vi "Versioned UI Post-Build Action.vi"(5 "Files Generated by Build":path[](array[path]), 6 "Top Level/Always Included VIs":path[](array[path]), 7 "Destination Path":path, 8 "error in (no error)":errorcluster, 9 "Target Name":string, 10 "Build Specification Name":string, 11 "Project Path":path) -> (0 "error out":errorcluster)   [LabVIEW 2021, in "CIF Build Actions.lvlib"]
uses:
  CIF Build Actions.lvlib
  <vilib>/regexp/Match Regular Expression.xnode
  CIFConfigurationFile/CIF Configuration File.lvlib
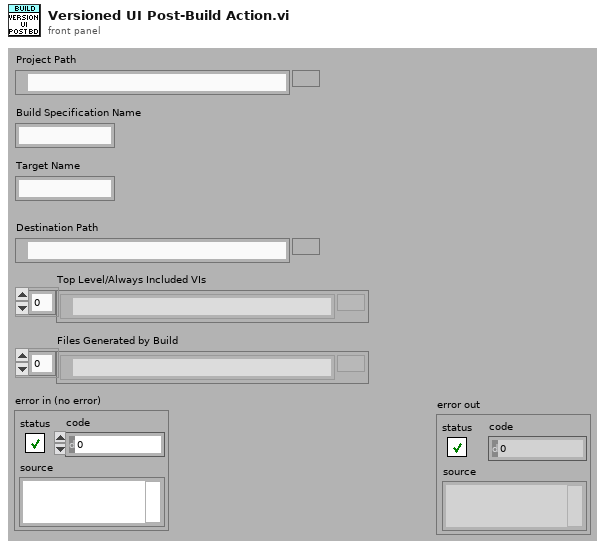
[diagram p1: front panel]
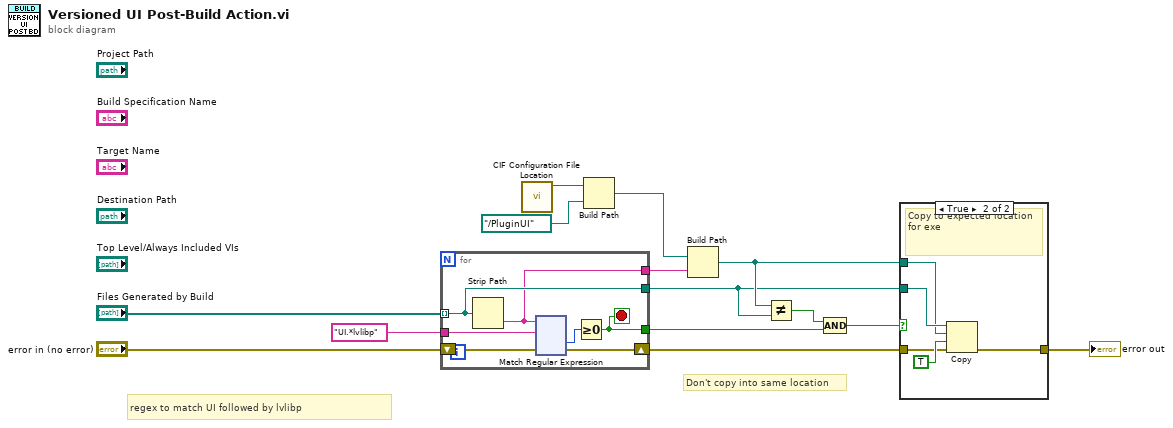
[diagram p0: block diagram]
diagram:
  # "Don't copy into same location"
  # "regex to match UI followed by lvlibp"
  n1 = for {
    tunnel: "Files Generated by Build" -> [w20] mode=indexing
    tunnel: "UI.*lvlibp" ("pattern") -> [w21]
    tunnel: [w20] -> w4
    tunnel: [w18] -> w10
    shift-right: [w16] -> w7
    shift-left: "error in (no error)" -> [w17]
    tunnel: [w15] -> w3
    stop <- w15 stop-if-true
    n2 = Strip Path(path=w20) -> (name=w18:string)  [unwired: 1 out]
    n3 = xnode "Match Regular Expression"("input string"=w18, "regular expression"=w21, "error in"=w17) -> ("offset past match"=w19:i32, "error out"=w16:errorcluster)  [unwired: 3 in, 3 out]
    n4 = Greater Or Equal To 0?(x=w19) -> (x >= 0?=w15:bool)
  }
  n5 = call "CIF Configuration File Location.vi"() -> ("configuration file path"=w14:path)  [unwired: 11 in]
  n6 = Build Path(base path=w14, name or relative path=path "../PluginUI") -> (appended path=w9:path)
  n7 = Build Path(base path=w9, name or relative path=w10) -> (appended path=w5:path)
  n8 = Not Equal?(x=w5, y=w4) -> (x != y?=w2:bool)
  n9 = Compound Arithmetic op=AND(w2, w3) -> (w1:bool)
  n10 = case shown="True" w1 {
    tunnel: w4 -> [_ w144]
    tunnel: w5 -> [_ w143]
    tunnel: w7 -> [w139 w141]
    tunnel: [w139 w140] -> w6
    frame False {
      # "PPL not found, could provide error"
    }
    frame True {
      # "Copy to expected location for exe"
      n11 = Copy(8:w141, 9:TRUE ("overwrite (F)"), 10:w143, 11:w144) -> (0:w140:errorcluster)  [unwired: 1 in, 2 out]
    }
  }
  "error out" <- w6
